vi "Parse XML String for Multiple Nodes.vi"() -> ()   [LabVIEW 2013]
doc: "This example demonstrates how to query an XML document by using an XPath expression and returns all the nodes that match the XPath expression."
uses:
  <vilib>/xml/Load XML String.vi
  <vilib>/xml/Close Reference(Node).vi
  <resource>/objmgr/DOMUserDefRef.rc
  <vilib>/xml/NI_XML.lvlib
panel:
  in  "XPath Expression":string="descendant::*"
  in  "XML String":string="<?xml version=\"1.0\" encoding=\"UTF-8\" standalone=\"no\" ?><office:document-content office:version=\"1.2\" xmlns:calcext=\"urn:org:documentfoundation:names:experimental:calc:xmlns:calcext:1.0\" xmlns:chart=\"urn:oasis:names:tc:opendocument:xmlns:chart:1.0\" xmlns:css3t=\"http://www.w3.org/TR/css3-text/\" xmlns:dc=\"http://purl.org/dc/elements/1.1/\" xmlns:dom=\"http://www.w3.org/2001/xml-events\" xmlns:dr3d=\"urn:oasis:names:tc:opendocument:xmlns:dr3d:1.0\" xmlns:draw=\"urn:oasis:names:tc:opendocument:xmlns:drawing:1.0\" xmlns:drawooo=\"http://openoffice.org/2010/draw\" xmlns:field=\"urn:openoffice:names:experimental:ooo-ms-interop:xmlns:field:1.0\" xmlns:fo=\"urn:oasis:names:tc:opendocument:xmlns:xsl-fo-compatible:1.0\" xmlns:form=\"urn:oasis:names:tc:opendocument:xmlns:form:1.0\" xmlns:formx=\"urn:openoffice:names:experimental:ooxml-odf-interop:xmlns:form:1.0\" xmlns:grddl=\"http://www.w3.org/2003/g/data-view#\" xmlns:loext=\"urn:org:documentfoundation:names:experimental:office:xmlns:loext:1.0\" xmlns:math=\"http://www.w3.org/1998/Math/MathML\" xmlns:meta=\"urn:oasis:names:tc:opendocument:xmlns:meta:1.0\" xmlns:number=\"urn:oasis:names:tc:opendocument:xmlns:datastyle:1.0\" xmlns:of=\"urn:oasis:names:tc:opendocument:xmlns:of:1.2\" xmlns:office=\"urn:oasis:names:tc:opendocument:xmlns:office:1.0\" xmlns:ooo=\"http://openoffice.org/2004/office\" xmlns:oooc=\"http://openoffice.org/2004/calc\" xmlns:ooow=\"http://openoffice.org/2004/writer\" xmlns:presentation=\"urn:oasis:names:tc:opendocument:xmlns:presentation:1.0\" xmlns:rpt=\"http://openoffice.org/2005/report\" xmlns:script=\"urn:oasis:names:tc:opendocument:xmlns:script:1.0\" xmlns:style=\"urn:oasis:names:tc:opendocument:xmlns:style:1.0\" xmlns:svg=\"urn:oasis:names:tc:opendocument:xmlns:svg-compatible:1.0\" xmlns:table=\"urn:oasis:names:tc:opendocument:xmlns:table:1.0\" xmlns:tableooo=\"http://openoffice.org/2009/table\" xmlns:text=\"urn:oasis:names:tc:opendocument:xmlns:text:1.0\" xmlns:xforms=\"http://www.w3.org/2002/xforms\" xmlns:xhtml=\"http://www.w3.org/1999/xhtml\" xmlns:xlink=\"http://www.w3.org/1999/xlink\" xmlns:xsd=\"http://www.w3.org/2001/XMLSchema\" xmlns:xsi=\"http://www.w3.org/2001/XMLSchema-instance\"><office:scripts/><office:font-face-decls><style:font-face style:font-family-generic=\"swiss\" style:font-pitch=\"variable\" style:name=\"Arial\" svg:font-family=\"Arial\"/><style:font-face style:font-family-generic=\"system\" style:font-pitch=\"variable\" style:name=\"Mangal\" svg:font-family=\"Mangal\"/><style:font-face style:font-family-generic=\"system\" style:font-pitch=\"variable\" style:name=\"Microsoft YaHei\" svg:font-family=\"'Microsoft YaHei'\"/><style:font-face style:font-family-generic=\"system\" style:font-pitch=\"variable\" style:name=\"Segoe UI\" svg:font-family=\"'Segoe UI'\"/><style:font-face style:font-family-generic=\"system\" style:font-pitch=\"variable\" style:name=\"Tahoma\" svg:font-family=\"Tahoma\"/></office:font-face-decls><office:automatic-styles><style:style style:family=\"table-column\" style:name=\"co1\"><style:table-column-properties fo:break-before=\"auto\" style:column-width=\"2.258cm\"/></style:style><style:style style:family=\"table-column\" style:name=\"co2\"><style:table-column-properties fo:break-before=\"auto\" style:column-width=\"5.999cm\"/></style:style><style:style style:family=\"table-row\" style:name=\"ro1\"><style:table-row-properties fo:break-before=\"auto\" style:row-height=\"0.453cm\" style:use-optimal-row-height=\"true\"/></style:style><style:style style:family=\"table-row\" style:name=\"ro2\"><style:table-row-properties fo:break-before=\"auto\" style:row-height=\"0.473cm\" style:use-optimal-row-height=\"true\"/></style:style><style:style style:family=\"table\" style:master-page-name=\"Default\" style:name=\"ta1\"><style:table-properties style:writing-mode=\"lr-tb\" table:display=\"true\"/></style:style></office:automatic-styles><office:body><office:spreadsheet><table:table table:name=\"Sheet1\" table:style-name=\"ta1\"><table:table-column table:default-cell-style-name=\"Default\" table:style-name=\"co1\"/><table:table-column table:default-cell-style-name=\"Default\" table:style-name=\"co2\"/><table:table-column table:default-cell-style-name=\"Default\" table:number-columns-repeated=\"11\" table:style-name=\"co1\"/><table:table-row table:style-name=\"ro1\"><table:table-cell calcext:value-type=\"string\" office:value-type=\"string\"><text:p>Title1</text:p></table:table-cell><table:table-cell table:number-columns-repeated=\"12\"/></table:table-row><table:table-row table:style-name=\"ro2\"><table:table-cell/><table:table-cell calcext:value-type=\"string\" office:value-type=\"string\"><text:p>aaaaaaaaaaaaaaaaaaaaa</text:p></table:table-cell><table:table-cell table:number-columns-repeated=\"5\"/><table:table-cell calcext:value-type=\"string\" office:value-type=\"string\"><text:p>H2</text:p></table:table-cell><table:table-cell table:number-columns-repeated=\"5\"/></table:table-row><table:table-row table:style-name=\"ro2\"><table:table-cell/><table:table-cell calcext:value-type=\"string\" office:value-type=\"string\"><text:p>bbbbbbbbbbbbbbbbbbbbb</text:p></table:table-cell><table:table-cell table:number-columns-repeated=\"11\"/></table:table-row><table:table-row table:style-name=\"ro2\"><table:table-cell/><table:table-cell calcext:value-type=\"string\" office:value-type=\"string\"><text:p>ccccccccccccccccccccc</text:p></table:table-cell><table:table-cell table:number-columns-repeated=\"11\"/></table:table-row><table:table-row table:style-name=\"ro2\"><table:table-cell/><table:table-cell calcext:value-type=\"string\" office:value-type=\"string\"><text:p>ddddddddddddddddddddd</text:p></table:table-cell><table:table-cell table:number-columns-repeated=\"11\"/></table:table-row><table:table-row table:style-name=\"ro1\"><table:table-cell calcext:value-type=\"string\" office:value-type=\"string\"><text:p>Title2</text:p></table:table-cell><table:table-cell table:number-columns-repeated=\"12\"/></table:table-row><table:table-row table:style-name=\"ro2\"><table:table-cell/><table:table-cell calcext:value-type=\"string\" office:value-type=\"string\"><text:p>eeeeeeeeeeeeeeeeeeeee</text:p></table:table-cell><table:table-cell table:number-columns-repeated=\"11\"/></table:table-row><table:table-row table:style-name=\"ro2\"><table:table-cell/><table:table-cell calcext:value-type=\"string\" office:value-type=\"string\"><text:p>ffffffffffffffffffffffffffffffffffffffff</text:p></table:table-cell><table:table-cell table:number-columns-repeated=\"11\"/></table:table-row><table:table-row table:style-name=\"ro1\"><table:table-cell/><table:table-cell calcext:value-type=\"string\" office:value-type=\"string\"><text:p>ggggggggggggggggggggg</text:p></table:table-cell><table:table-cell table:number-columns-repeated=\"11\"/></table:table-row><table:table-row table:number-rows-repeated=\"5\" table:style-name=\"ro1\"><table:table-cell table:number-columns-repeated=\"13\"/></table:table-row><table:table-row table:style-name=\"ro1\"><table:table-cell table:number-columns-repeated=\"4\"/><table:table-cell calcext:value-type=\"string\" office:value-type=\"string\"><text:p>E16</text:p></table:table-cell><table:table-cell table:number-columns-repeated=\"8\"/></table:table-row><table:table-row table:number-rows-repeated=\"10\" table:style-name=\"ro1\"><table:table-cell table:number-columns-repeated=\"13\"/></table:table-row><table:table-row table:style-name=\"ro1\"><table:table-cell table:number-columns-repeated=\"12\"/><table:table-cell calcext:value-type=\"string\" office:value-type=\"string\"><text:p>M26</text:p></table:table-cell></table:table-row></table:table><table:named-expressions/></office:spreadsheet></office:body></office:document-content>"
  out "Search Results":string[](array[string])=["<office:scripts/>", "<office:font-face-decls><style:font-face style:font-family-generic=\"swiss\" style:font-pitch=\"variable\" style:name=\"Arial\" svg:font-family=\"Arial\"/><style:font-face style:font-family-generic=\"system\" style:font-pitch=\"variable\" style:name=\"Mangal\" svg:font-family=\"Mangal\"/><style:font-face style:font-family-generic=\"system\" style:font-pitch=\"variable\" style:name=\"Microsoft YaHei\" svg:font-family=\"'Microsoft YaHei'\"/><style:font-face style:font-family-generic=\"system\" style:font-pitch=\"variable\" style:name=\"Segoe UI\" svg:font-family=\"'Segoe UI'\"/><style:font-face style:font-family-generic=\"system\" style:font-pitch=\"variable\" style:name=\"Tahoma\" svg:font-family=\"Tahoma\"/></office:font-face-decls>", "<style:font-face style:font-family-generic=\"swiss\" style:font-pitch=\"variable\" style:name=\"Arial\" svg:font-family=\"Arial\"/>", "<style:font-face style:font-family-generic=\"system\" style:font-pitch=\"variable\" style:name=\"Mangal\" svg:font-family=\"Mangal\"/>", "<style:font-face style:font-family-generic=\"system\" style:font-pitch=\"variable\" style:name=\"Microsoft YaHei\" svg:font-family=\"'Microsoft YaHei'\"/>", "<style:font-face style:font-family-generic=\"system\" style:font-pitch=\"variable\" style:name=\"Segoe UI\" svg:font-family=\"'Segoe UI'\"/>", "<style:font-face style:font-family-generic=\"system\" style:font-pitch=\"variable\" style:name=\"Tahoma\" svg:font-family=\"Tahoma\"/>", "<office:automatic-styles><style:style style:family=\"table-column\" style:name=\"co1\"><style:table-column-properties fo:break-before=\"auto\" style:column-width=\"2.258cm\"/></style:style><style:style style:family=\"table-column\" style:name=\"co2\"><style:table-column-properties fo:break-before=\"auto\" style:column-width=\"5.999cm\"/></style:style><style:style style:family=\"table-row\" style:name=\"ro1\"><style:table-row-properties fo:break-before=\"auto\" style:row-height=\"0.453cm\" style:use-optimal-row-height=\"true\"/></style:style><style:style style:family=\"table-row\" style:name=\"ro2\"><style:table-row-properties fo:break-before=\"auto\" style:row-height=\"0.473cm\" style:use-optimal-row-height=\"true\"/></style:style><style:style style:family=\"table\" style:master-page-name=\"Default\" style:name=\"ta1\"><style:table-properties style:writing-mode=\"lr-tb\" table:display=\"true\"/></style:style></office:automatic-styles>", "<style:style style:family=\"table-column\" style:name=\"co1\"><style:table-column-properties fo:break-before=\"auto\" style:column-width=\"2.258cm\"/></style:style>", "<style:table-column-properties fo:break-before=\"auto\" style:column-width=\"2.258cm\"/>", "<style:style style:family=\"table-column\" style:name=\"co2\"><style:table-column-properties fo:break-before=\"auto\" style:column-width=\"5.999cm\"/></style:style>", "<style:table-column-properties fo:break-before=\"auto\" style:column-width=\"5.999cm\"/>", "<style:style style:family=\"table-row\" style:name=\"ro1\"><style:table-row-properties fo:break-before=\"auto\" style:row-height=\"0.453cm\" style:use-optimal-row-height=\"true\"/></style:style>", "<style:table-row-properties fo:break-before=\"auto\" style:row-height=\"0.453cm\" style:use-optimal-row-height=\"true\"/>", "<style:style style:family=\"table-row\" style:name=\"ro2\"><style:table-row-properties fo:break-before=\"auto\" style:row-height=\"0.473cm\" style:use-optimal-row-height=\"true\"/></style:style>", "<style:table-row-properties fo:break-before=\"auto\" style:row-height=\"0.473cm\" style:use-optimal-row-height=\"true\"/>", "<style:style style:family=\"table\" style:master-page-name=\"Default\" style:name=\"ta1\"><style:table-properties style:writing-mode=\"lr-tb\" table:display=\"true\"/></style:style>", "<style:table-properties style:writing-mode=\"lr-tb\" table:display=\"true\"/>", "<office:body><office:spreadsheet><table:table table:name=\"Sheet1\" table:style-name=\"ta1\"><table:table-column table:default-cell-style-name=\"Default\" table:style-name=\"co1\"/><table:table-column table:default-cell-style-name=\"Default\" table:style-name=\"co2\"/><table:table-column table:default-cell-style-name=\"Default\" table:number-columns-repeated=\"11\" table:style-name=\"co1\"/><table:table-row table:style-name=\"ro1\"><table:table-cell calcext:value-type=\"string\" office:value-type=\"string\"><text:p>Title1</text:p></table:table-cell><table:table-cell table:number-columns-repeated=\"12\"/></table:table-row><table:table-row table:style-name=\"ro2\"><table:table-cell/><table:table-cell calcext:value-type=\"string\" office:value-type=\"string\"><text:p>aaaaaaaaaaaaaaaaaaaaa</text:p></table:table-cell><table:table-cell table:number-columns-repeated=\"5\"/><table:table-cell calcext:value-type=\"string\" office:value-type=\"string\"><text:p>H2</text:p></table:table-cell><table:table-cell table:number-columns-repeated=\"5\"/></table:table-row><table:table-row table:style-name=\"ro2\"><table:table-cell/><table:table-cell calcext:value-type=\"string\" office:value-type=\"string\"><text:p>bbbbbbbbbbbbbbbbbbbbb</text:p></table:table-cell><table:table-cell table:number-columns-repeated=\"11\"/></table:table-row><table:table-row table:style-name=\"ro2\"><table:table-cell/><table:table-cell calcext:value-type=\"string\" office:value-type=\"string\"><text:p>ccccccccccccccccccccc</text:p></table:table-cell><table:table-cell table:number-columns-repeated=\"11\"/></table:table-row><table:table-row table:style-name=\"ro2\"><table:table-cell/><table:table-cell calcext:value-type=\"string\" office:value-type=\"string\"><text:p>ddddddddddddddddddddd</text:p></table:table-cell><table:table-cell table:number-columns-repeated=\"11\"/></table:table-row><table:table-row table:style-name=\"ro1\"><table:table-cell calcext:value-type=\"string\" office:value-type=\"string\"><text:p>Title2</text:p></table:table-cell><table:table-cell table:number-columns-repeated=\"12\"/></table:table-row><table:table-row table:style-name=\"ro2\"><table:table-cell/><table:table-cell calcext:value-type=\"string\" office:value-type=\"string\"><text:p>eeeeeeeeeeeeeeeeeeeee</text:p></table:table-cell><table:table-cell table:number-columns-repeated=\"11\"/></table:table-row><table:table-row table:style-name=\"ro2\"><table:table-cell/><table:table-cell calcext:value-type=\"string\" office:value-type=\"string\"><text:p>ffffffffffffffffffffffffffffffffffffffff</text:p></table:table-cell><table:table-cell table:number-columns-repeated=\"11\"/></table:table-row><table:table-row table:style-name=\"ro1\"><table:table-cell/><table:table-cell calcext:value-type=\"string\" office:value-type=\"string\"><text:p>ggggggggggggggggggggg</text:p></table:table-cell><table:table-cell table:number-columns-repeated=\"11\"/></table:table-row><table:table-row table:number-rows-repeated=\"5\" table:style-name=\"ro1\"><table:table-cell table:number-columns-repeated=\"13\"/></table:table-row><table:table-row table:style-name=\"ro1\"><table:table-cell table:number-columns-repeated=\"4\"/><table:table-cell calcext:value-type=\"string\" office:value-type=\"string\"><text:p>E16</text:p></table:table-cell><table:table-cell table:number-columns-repeated=\"8\"/></table:table-row><table:table-row table:number-rows-repeated=\"10\" table:style-name=\"ro1\"><table:table-cell table:number-columns-repeated=\"13\"/></table:table-row><table:table-row table:style-name=\"ro1\"><table:table-cell table:number-columns-repeated=\"12\"/><table:table-cell calcext:value-type=\"string\" office:value-type=\"string\"><text:p>M26</text:p></table:table-cell></table:table-row></table:table><table:named-expressions/></office:spreadsheet></office:body>", "<office:spreadsheet><table:table table:name=\"Sheet1\" table:style-name=\"ta1\"><table:table-column table:default-cell-style-name=\"Default\" table:style-name=\"co1\"/><table:table-column table:default-cell-style-name=\"Default\" table:style-name=\"co2\"/><table:table-column table:default-cell-style-name=\"Default\" table:number-columns-repeated=\"11\" table:style-name=\"co1\"/><table:table-row table:style-name=\"ro1\"><table:table-cell calcext:value-type=\"string\" office:value-type=\"string\"><text:p>Title1</text:p></table:table-cell><table:table-cell table:number-columns-repeated=\"12\"/></table:table-row><table:table-row table:style-name=\"ro2\"><table:table-cell/><table:table-cell calcext:value-type=\"string\" office:value-type=\"string\"><text:p>aaaaaaaaaaaaaaaaaaaaa</text:p></table:table-cell><table:table-cell table:number-columns-repeated=\"5\"/><table:table-cell calcext:value-type=\"string\" office:value-type=\"string\"><text:p>H2</text:p></table:table-cell><table:table-cell table:number-columns-repeated=\"5\"/></table:table-row><table:table-row table:style-name=\"ro2\"><table:table-cell/><table:table-cell calcext:value-type=\"string\" office:value-type=\"string\"><text:p>bbbbbbbbbbbbbbbbbbbbb</text:p></table:table-cell><table:table-cell table:number-columns-repeated=\"11\"/></table:table-row><table:table-row table:style-name=\"ro2\"><table:table-cell/><table:table-cell calcext:value-type=\"string\" office:value-type=\"string\"><text:p>ccccccccccccccccccccc</text:p></table:table-cell><table:table-cell table:number-columns-repeated=\"11\"/></table:table-row><table:table-row table:style-name=\"ro2\"><table:table-cell/><table:table-cell calcext:value-type=\"string\" office:value-type=\"string\"><text:p>ddddddddddddddddddddd</text:p></table:table-cell><table:table-cell table:number-columns-repeated=\"11\"/></table:table-row><table:table-row table:style-name=\"ro1\"><table:table-cell calcext:value-type=\"string\" office:value-type=\"string\"><text:p>Title2</text:p></table:table-cell><table:table-cell table:number-columns-repeated=\"12\"/></table:table-row><table:table-row table:style-name=\"ro2\"><table:table-cell/><table:table-cell calcext:value-type=\"string\" office:value-type=\"string\"><text:p>eeeeeeeeeeeeeeeeeeeee</text:p></table:table-cell><table:table-cell table:number-columns-repeated=\"11\"/></table:table-row><table:table-row table:style-name=\"ro2\"><table:table-cell/><table:table-cell calcext:value-type=\"string\" office:value-type=\"string\"><text:p>ffffffffffffffffffffffffffffffffffffffff</text:p></table:table-cell><table:table-cell table:number-columns-repeated=\"11\"/></table:table-row><table:table-row table:style-name=\"ro1\"><table:table-cell/><table:table-cell calcext:value-type=\"string\" office:value-type=\"string\"><text:p>ggggggggggggggggggggg</text:p></table:table-cell><table:table-cell table:number-columns-repeated=\"11\"/></table:table-row><table:table-row table:number-rows-repeated=\"5\" table:style-name=\"ro1\"><table:table-cell table:number-columns-repeated=\"13\"/></table:table-row><table:table-row table:style-name=\"ro1\"><table:table-cell table:number-columns-repeated=\"4\"/><table:table-cell calcext:value-type=\"string\" office:value-type=\"string\"><text:p>E16</text:p></table:table-cell><table:table-cell table:number-columns-repeated=\"8\"/></table:table-row><table:table-row table:number-rows-repeated=\"10\" table:style-name=\"ro1\"><table:table-cell table:number-columns-repeated=\"13\"/></table:table-row><table:table-row table:style-name=\"ro1\"><table:table-cell table:number-columns-repeated=\"12\"/><table:table-cell calcext:value-type=\"string\" office:value-type=\"string\"><text:p>M26</text:p></table:table-cell></table:table-row></table:table><table:named-expressions/></office:spreadsheet>", "<table:table table:name=\"Sheet1\" table:style-name=\"ta1\"><table:table-column table:default-cell-style-name=\"Default\" table:style-name=\"co1\"/><table:table-column table:default-cell-style-name=\"Default\" table:style-name=\"co2\"/><table:table-column table:default-cell-style-name=\"Default\" table:number-columns-repeated=\"11\" table:style-name=\"co1\"/><table:table-row table:style-name=\"ro1\"><table:table-cell calcext:value-type=\"string\" office:value-type=\"string\"><text:p>Title1</text:p></table:table-cell><table:table-cell table:number-columns-repeated=\"12\"/></table:table-row><table:table-row table:style-name=\"ro2\"><table:table-cell/><table:table-cell calcext:value-type=\"string\" office:value-type=\"string\"><text:p>aaaaaaaaaaaaaaaaaaaaa</text:p></table:table-cell><table:table-cell table:number-columns-repeated=\"5\"/><table:table-cell calcext:value-type=\"string\" office:value-type=\"string\"><text:p>H2</text:p></table:table-cell><table:table-cell table:number-columns-repeated=\"5\"/></table:table-row><table:table-row table:style-name=\"ro2\"><table:table-cell/><table:table-cell calcext:value-type=\"string\" office:value-type=\"string\"><text:p>bbbbbbbbbbbbbbbbbbbbb</text:p></table:table-cell><table:table-cell table:number-columns-repeated=\"11\"/></table:table-row><table:table-row table:style-name=\"ro2\"><table:table-cell/><table:table-cell calcext:value-type=\"string\" office:value-type=\"string\"><text:p>ccccccccccccccccccccc</text:p></table:table-cell><table:table-cell table:number-columns-repeated=\"11\"/></table:table-row><table:table-row table:style-name=\"ro2\"><table:table-cell/><table:table-cell calcext:value-type=\"string\" office:value-type=\"string\"><text:p>ddddddddddddddddddddd</text:p></table:table-cell><table:table-cell table:number-columns-repeated=\"11\"/></table:table-row><table:table-row table:style-name=\"ro1\"><table:table-cell calcext:value-type=\"string\" office:value-type=\"string\"><text:p>Title2</text:p></table:table-cell><table:table-cell table:number-columns-repeated=\"12\"/></table:table-row><table:table-row table:style-name=\"ro2\"><table:table-cell/><table:table-cell calcext:value-type=\"string\" office:value-type=\"string\"><text:p>eeeeeeeeeeeeeeeeeeeee</text:p></table:table-cell><table:table-cell table:number-columns-repeated=\"11\"/></table:table-row><table:table-row table:style-name=\"ro2\"><table:table-cell/><table:table-cell calcext:value-type=\"string\" office:value-type=\"string\"><text:p>ffffffffffffffffffffffffffffffffffffffff</text:p></table:table-cell><table:table-cell table:number-columns-repeated=\"11\"/></table:table-row><table:table-row table:style-name=\"ro1\"><table:table-cell/><table:table-cell calcext:value-type=\"string\" office:value-type=\"string\"><text:p>ggggggggggggggggggggg</text:p></table:table-cell><table:table-cell table:number-columns-repeated=\"11\"/></table:table-row><table:table-row table:number-rows-repeated=\"5\" table:style-name=\"ro1\"><table:table-cell table:number-columns-repeated=\"13\"/></table:table-row><table:table-row table:style-name=\"ro1\"><table:table-cell table:number-columns-repeated=\"4\"/><table:table-cell calcext:value-type=\"string\" office:value-type=\"string\"><text:p>E16</text:p></table:table-cell><table:table-cell table:number-columns-repeated=\"8\"/></table:table-row><table:table-row table:number-rows-repeated=\"10\" table:style-name=\"ro1\"><table:table-cell table:number-columns-repeated=\"13\"/></table:table-row><table:table-row table:style-name=\"ro1\"><table:table-cell table:number-columns-repeated=\"12\"/><table:table-cell calcext:value-type=\"string\" office:value-type=\"string\"><text:p>M26</text:p></table:table-cell></table:table-row></table:table>", "<table:table-column table:default-cell-style-name=\"Default\" table:style-name=\"co1\"/>", "<table:table-column table:default-cell-style-name=\"Default\" table:style-name=\"co2\"/>", "<table:table-column table:default-cell-style-name=\"Default\" table:number-columns-repeated=\"11\" table:style-name=\"co1\"/>", "<table:table-row table:style-name=\"ro1\"><table:table-cell calcext:value-type=\"string\" office:value-type=\"string\"><text:p>Title1</text:p></table:table-cell><table:table-cell table:number-columns-repeated=\"12\"/></table:table-row>", "<table:table-cell calcext:value-type=\"string\" office:value-type=\"string\"><text:p>Title1</text:p></table:table-cell>", "<text:p>Title1</text:p>", "<table:table-cell table:number-columns-repeated=\"12\"/>", "<table:table-row table:style-name=\"ro2\"><table:table-cell/><table:table-cell calcext:value-type=\"string\" office:value-type=\"string\"><text:p>aaaaaaaaaaaaaaaaaaaaa</text:p></table:table-cell><table:table-cell table:number-columns-repeated=\"5\"/><table:table-cell calcext:value-type=\"string\" office:value-type=\"string\"><text:p>H2</text:p></table:table-cell><table:table-cell table:number-columns-repeated=\"5\"/></table:table-row>", "<table:table-cell/>", "<table:table-cell calcext:value-type=\"string\" office:value-type=\"string\"><text:p>aaaaaaaaaaaaaaaaaaaaa</text:p></table:table-cell>", "<text:p>aaaaaaaaaaaaaaaaaaaaa</text:p>", "<table:table-cell table:number-columns-repeated=\"5\"/>", "<table:table-cell calcext:value-type=\"string\" office:value-type=\"string\"><text:p>H2</text:p></table:table-cell>", "<text:p>H2</text:p>", "<table:table-cell table:number-columns-repeated=\"5\"/>", "<table:table-row table:style-name=\"ro2\"><table:table-cell/><table:table-cell calcext:value-type=\"string\" office:value-type=\"string\"><text:p>bbbbbbbbbbbbbbbbbbbbb</text:p></table:table-cell><table:table-cell table:number-columns-repeated=\"11\"/></table:table-row>", "<table:table-cell/>", "<table:table-cell calcext:value-type=\"string\" office:value-type=\"string\"><text:p>bbbbbbbbbbbbbbbbbbbbb</text:p></table:table-cell>", "<text:p>bbbbbbbbbbbbbbbbbbbbb</text:p>", "<table:table-cell table:number-columns-repeated=\"11\"/>", "<table:table-row table:style-name=\"ro2\"><table:table-cell/><table:table-cell calcext:value-type=\"string\" office:value-type=\"string\"><text:p>ccccccccccccccccccccc</text:p></table:table-cell><table:table-cell table:number-columns-repeated=\"11\"/></table:table-row>", "<table:table-cell/>", "<table:table-cell calcext:value-type=\"string\" office:value-type=\"string\"><text:p>ccccccccccccccccccccc</text:p></table:table-cell>", "<text:p>ccccccccccccccccccccc</text:p>", "<table:table-cell table:number-columns-repeated=\"11\"/>", "<table:table-row table:style-name=\"ro2\"><table:table-cell/><table:table-cell calcext:value-type=\"string\" office:value-type=\"string\"><text:p>ddddddddddddddddddddd</text:p></table:table-cell><table:table-cell table:number-columns-repeated=\"11\"/></table:table-row>", "<table:table-cell/>", "<table:table-cell calcext:value-type=\"string\" office:value-type=\"string\"><text:p>ddddddddddddddddddddd</text:p></table:table-cell>", "<text:p>ddddddddddddddddddddd</text:p>", "<table:table-cell table:number-columns-repeated=\"11\"/>", "<table:table-row table:style-name=\"ro1\"><table:table-cell calcext:value-type=\"string\" office:value-type=\"string\"><text:p>Title2</text:p></table:table-cell><table:table-cell table:number-columns-repeated=\"12\"/></table:table-row>", "<table:table-cell calcext:value-type=\"string\" office:value-type=\"string\"><text:p>Title2</text:p></table:table-cell>", "<text:p>Title2</text:p>", "<table:table-cell table:number-columns-repeated=\"12\"/>", "<table:table-row table:style-name=\"ro2\"><table:table-cell/><table:table-cell calcext:value-type=\"string\" office:value-type=\"string\"><text:p>eeeeeeeeeeeeeeeeeeeee</text:p></table:table-cell><table:table-cell table:number-columns-repeated=\"11\"/></table:table-row>", "<table:table-cell/>", "<table:table-cell calcext:value-type=\"string\" office:value-type=\"string\"><text:p>eeeeeeeeeeeeeeeeeeeee</text:p></table:table-cell>", "<text:p>eeeeeeeeeeeeeeeeeeeee</text:p>", "<table:table-cell table:number-columns-repeated=\"11\"/>", "<table:table-row table:style-name=\"ro2\"><table:table-cell/><table:table-cell calcext:value-type=\"string\" office:value-type=\"string\"><text:p>ffffffffffffffffffffffffffffffffffffffff</text:p></table:table-cell><table:table-cell table:number-columns-repeated=\"11\"/></table:table-row>", "<table:table-cell/>", "<table:table-cell calcext:value-type=\"string\" office:value-type=\"string\"><text:p>ffffffffffffffffffffffffffffffffffffffff</text:p></table:table-cell>", "<text:p>ffffffffffffffffffffffffffffffffffffffff</text:p>", "<table:table-cell table:number-columns-repeated=\"11\"/>", "<table:table-row table:style-name=\"ro1\"><table:table-cell/><table:table-cell calcext:value-type=\"string\" office:value-type=\"string\"><text:p>ggggggggggggggggggggg</text:p></table:table-cell><table:table-cell table:number-columns-repeated=\"11\"/></table:table-row>", "<table:table-cell/>", "<table:table-cell calcext:value-type=\"string\" office:value-type=\"string\"><text:p>ggggggggggggggggggggg</text:p></table:table-cell>", "<text:p>ggggggggggggggggggggg</text:p>", "<table:table-cell table:number-columns-repeated=\"11\"/>", "<table:table-row table:number-rows-repeated=\"5\" table:style-name=\"ro1\"><table:table-cell table:number-columns-repeated=\"13\"/></table:table-row>", "<table:table-cell table:number-columns-repeated=\"13\"/>", "<table:table-row table:style-name=\"ro1\"><table:table-cell table:number-columns-repeated=\"4\"/><table:table-cell calcext:value-type=\"string\" office:value-type=\"string\"><text:p>E16</text:p></table:table-cell><table:table-cell table:number-columns-repeated=\"8\"/></table:table-row>", "<table:table-cell table:number-columns-repeated=\"4\"/>", "<table:table-cell calcext:value-type=\"string\" office:value-type=\"string\"><text:p>E16</text:p></table:table-cell>", "<text:p>E16</text:p>", "<table:table-cell table:number-columns-repeated=\"8\"/>", "<table:table-row table:number-rows-repeated=\"10\" table:style-name=\"ro1\"><table:table-cell table:number-columns-repeated=\"13\"/></table:table-row>", "<table:table-cell table:number-columns-repeated=\"13\"/>", "<table:table-row table:style-name=\"ro1\"><table:table-cell table:number-columns-repeated=\"12\"/><table:table-cell calcext:value-type=\"string\" office:value-type=\"string\"><text:p>M26</text:p></table:table-cell></table:table-row>", "<table:table-cell table:number-columns-repeated=\"12\"/>", "<table:table-cell calcext:value-type=\"string\" office:value-type=\"string\"><text:p>M26</text:p></table:table-cell>", "<text:p>M26</text:p>", "<table:named-expressions/>"]
  # "Overview: Demonstrates the use of the XML Parser VIs and functions to search an XML string for multiple nodes (tags) that match a given XPath search expression.\nInstructions:\nRun the VI."
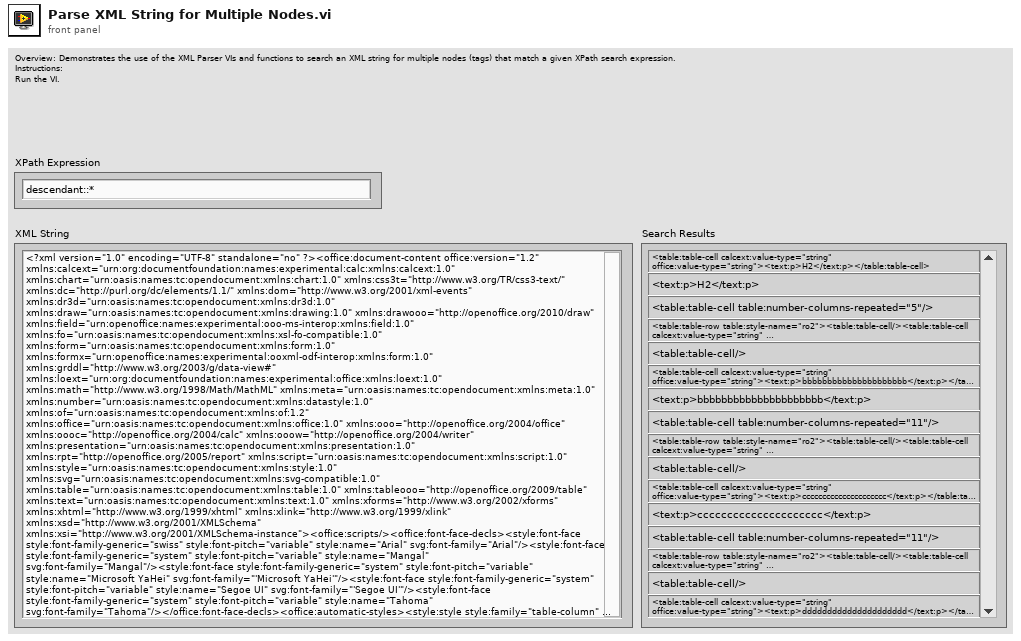
[diagram p1: front panel]
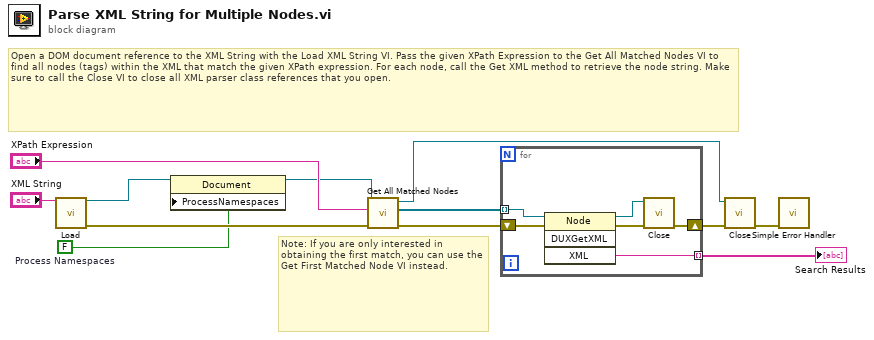
[diagram p0: block diagram]
diagram:
  w1 = FALSE  # Process Namespaces
  # "Note: If you are only interested in obtaining the first match, you can use the Get First Matched Node VI instead."
  # "Open a DOM document reference to the XML String with the Load XML String VI. Pass the given XPath Expression to the Get All Matched Nodes VI to find all nodes (tags) within the XML that match the given XPath expression. For each node, call the Get XML method to retrieve the node string. Make sure to call the Close VI to close all XML parser class references that you open."
  n1 = call-poly <vilib>:"Load.vi"("XML string"="XML String") -> ("DOM document out"=w4:refnum<k20>, "error out"=w3:errorcluster)  [unwired: 12 in, 1 out]
  n2 = property class="Document"(reference=w4, "ProcessNamespaces"=w1) -> (reference out=w2:refnum<k20>)  [unwired: 1 in, 1 out]
  n3 = call <vilib>:"Get All Matched Nodes.vi"("error in (no error)"=w3, "XPath expression"="XPath Expression", "node in"=w2) -> ("error out"=w11:errorcluster, "node result array"=w12:refnum<k20>[], "node out"=w8:refnum<k20>)  [unwired: 6 out]
  n4 = for {
    tunnel: w12 -> [w14] mode=indexing
    shift-right: [w16] -> w9
    shift-left: w11 -> [w15]
    tunnel: [w13] -> w6 mode=indexing
    n5 = invoke on="Invoke Node" class="Node" method="DUXGetXML"(reference=w14, error in=w15) -> (reference out=w17:refnum<k20>, error out=w18:errorcluster, "XML"=w13:string)  [unwired: 2 in, 1 out]
    n6 = call-poly <vilib>:"Close.vi"("error in (no error)"=w18, "node"=w17) -> ("error out"=w16:errorcluster)  [unwired: 7 out]
  }
  "Search Results" <- w6
  n7 = call-poly <vilib>:"Close.vi"("error in (no error)"=w9, "node"=w8) -> ("error out"=w7:errorcluster)  [unwired: 7 out]
  n8 = call <vilib>:"Simple Error Handler.vi"("error in (no error)"=w7) -> ()  [unwired: 1 in, 8 out]
